vi "Get Data Name from TD__ogtk.vi"(8 "error in (no error)":errorcluster, 10 "Type Descriptor":T1) -> (0 "error":errorcluster, 2 "name":string)   [LabVIEW 2020, in "openg_variant.lvlib"]
doc: "Returns the name of the data described by the type string input."
uses:
  openg_variant.lvlib
  Type Descriptor__ogtk.ctl
  openg_error.lvlib
panel:
  # "[OpenG VI Tags] ***Do Not Remove***"
  # "Get Data Name from TD.vi\n\nReturns the name of the data described by the type string input.\n\nPlease visit http://www.OpenG.org to learn about the\nOpen Source LabVIEW software movement.\n\nNOTICE -- YOU MUST LEAVE THIS NOTICE IN PLACE.  PER THE TERMS OF THE LICENSE BELOW, YOU MAY SUBLICENSE THIS SOFTWARE \nIN ANY WAY THAT DOES NOT CONFLICT WITH THIS LICENSE.\n\n### BSD License (http://www.opensource.org/licenses/bsd-license.php) Begin ###\n \nCopyright (c) 2002, Jean-Pierre Drolet <drolet_jp@hotmail.com>\nCopyright (c) 2002-2006, Jim Kring <jim@jimkring.com>\n\nAll rights reserved.\n\nRedistribution and use in source and binary forms, with or without modification, are permitted provided that the following conditions are met:\n\n    * Redistributions of source code must retain the above copyright notice, this list of conditions and the following disclaimer.\n    * Redistributions in binary form must reproduce the above copyright notice, this list of conditions and the following disclaimer in the \n       documentation and/or other materials provided with the distribution.\n    * Neither the name of SciWare, James Kring, Inc., nor the names of its contributors may be used to endorse or promote products derived \n       from this software without specific prior written permission.\n\nTHIS SOFTWARE IS PROVIDED BY THE COPYRIGHT HOLDERS AND CONTRIBUTORS \"AS IS\" AND ANY EXPRESS OR IMPLIED WARRANTIES, \nINCLUDING, BUT NOT LIMITED TO, THE IMPLIED WARRANTIES OF MERCHANTABILITY AND FITNESS FOR A PARTICULAR PURPOSE ARE \nDISCLAIMED. IN NO EVENT SHALL THE COPYRIGHT OWNER OR CONTRIBUTORS BE LIABLE FOR ANY DIRECT, INDIRECT, INCIDENTAL,\n SPECIAL, EXEMPLARY, OR CONSEQUENTIAL DAMAGES (INCLUDING, BUT NOT LIMITED TO, PROCUREMENT OF SUBSTITUTE GOODS OR \nSERVICES; LOSS OF USE, DATA, OR PROFITS; OR BUSINESS INTERRUPTION) HOWEVER CAUSED AND ON ANY THEORY OF LIABILITY, \nWHETHER IN CONTRACT, STRICT LIABILITY, OR TORT (INCLUDING NEGLIGENCE OR OTHERWISE) ARISING IN ANY WAY OUT OF THE USE \nOF THIS SOFTWARE, EVEN IF ADVISED OF THE POSSIBILITY OF SUCH DAMAGE.\n\n### BSD License End ###"
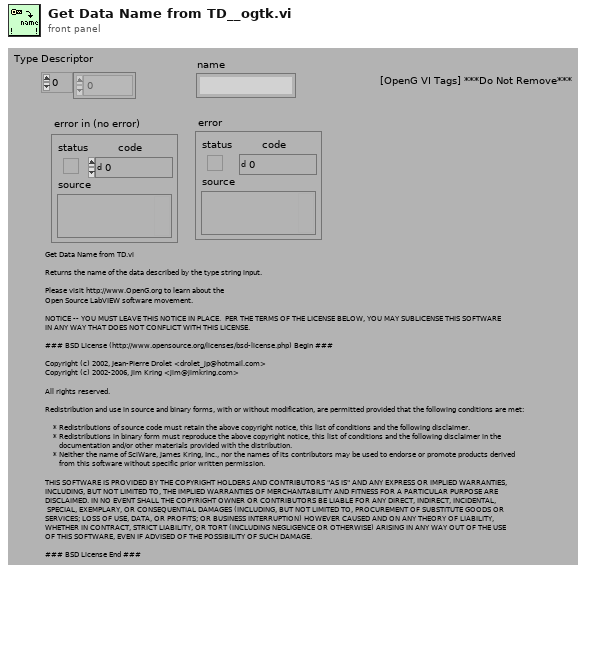
[diagram p1: front panel]
types:
  T1 = typedef "openg_variant.lvlib/Type Descriptor__ogtk.ctl" = i16[]
  T2 = typedef "openg_variant.lvlib/Type Descriptor Header__ogtk.ctl" = cluster{"length":u16, "private":u8, "type":T3, "# elements":u16}
  T3 = typedef "openg_variant.lvlib/Type Descriptor Enumeration__ogtk.ctl" = enum8{"<Null>", "I8", "I16", "I32", "I64", "U8", "U16", "U32", "U64", "SGL", "DBL", "EXT", "CSG", "CDB", "CXT", "0x0F", "0x10", "0x11", "0x12", "0x13", "0x14", "Enum U8", "Enum U16", "Enum U32", "Enum U64", "SGL PQ", "DBL PQ", "EXT PQ", "CSG PQ", "CDB PQ", "CXT PQ", "0x1F", "0x20", "Boolean", "0x22", "0x23", "0x24", "0x25", "0x26", "0x27", "0x28", "0x29", "0x2A", "0x2B", "0x2C", "0x2D", "0x2E", "0x2F", "String", "0x31", "Path", "Pict", "0x34", "0x35", "0x36", "DAQ", "0x38", "0x39", "0x3A", "0x3B", "0x3C", "0x3D", "0x3E", "0x3F", "Array", "0x41", "0x42", "0x43", "0x44", "0x45", "0x46", "0x47", "0x48", "0x49", "0x4A", "0x4B", "0x4C", "0x4D", "0x4E", "0x4F", "Cluster", "0x51", "0x52", "Variant", "Waveform", "0x55", "0x56", "0x57", "0x58", "0x59", "0x5A", "0x5B", "0x5C", "0x5D", "0x5E", "Fixed Point", "0x60", "0x61", "0x62", "0x63", "0x64", "0x65", "0x66", "0x67", "0x68", "0x69", "0x6A", "0x6B", "0x6C", "0x6D", "0x6E", "0x6F", "Refnum", "0x71", "0x72", "Set Collection", "Map Collection"}
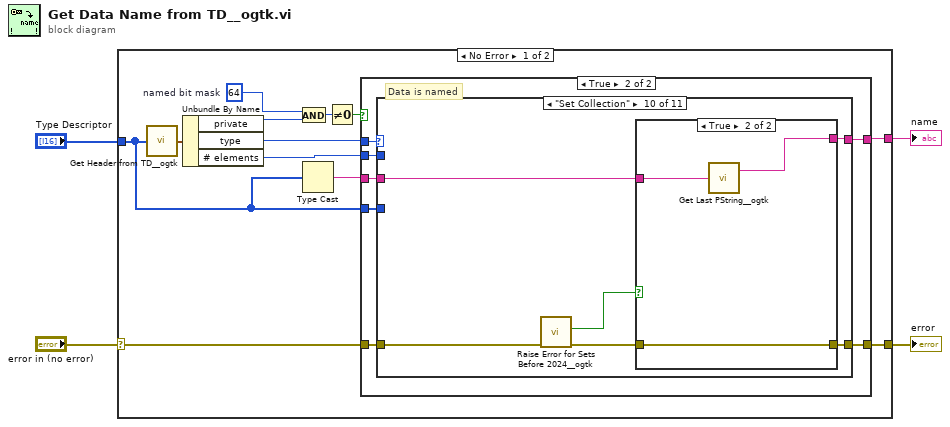
[diagram p0: block diagram]
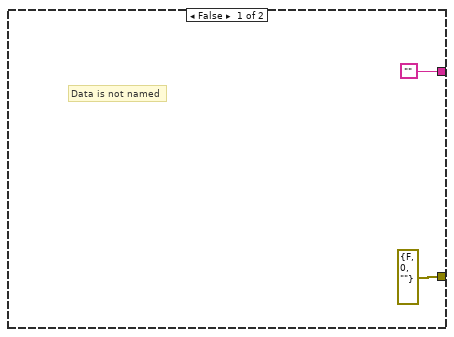
[diagram p2: hidden frame]
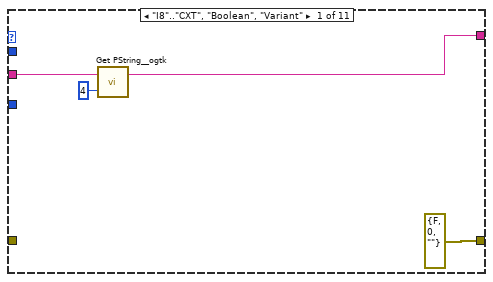
[diagram p3: hidden frame]
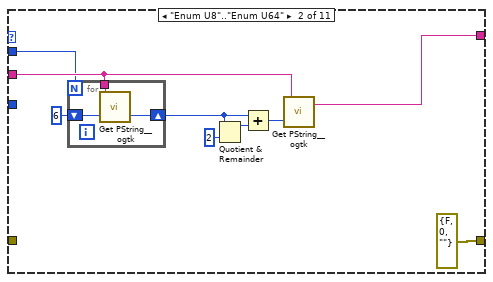
[diagram p4: hidden frame]
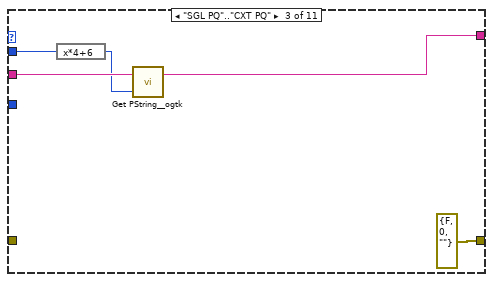
[diagram p5: hidden frame]
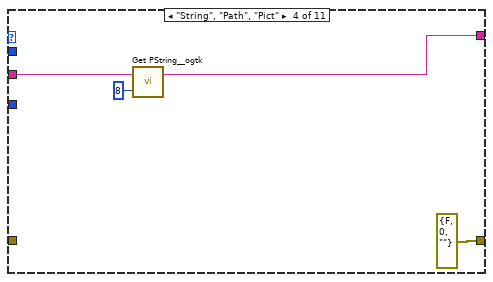
[diagram p6: hidden frame]
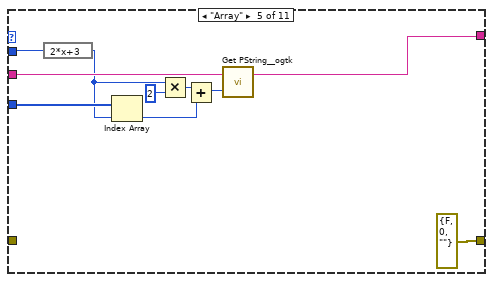
[diagram p7: hidden frame]
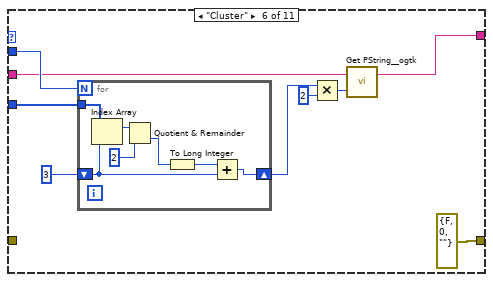
[diagram p8: hidden frame]
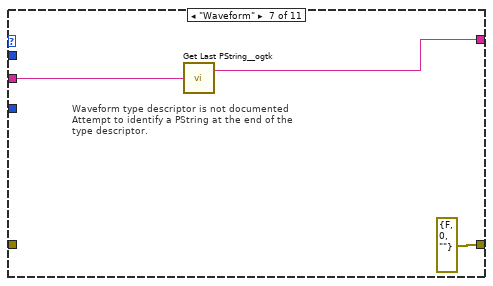
[diagram p9: hidden frame]
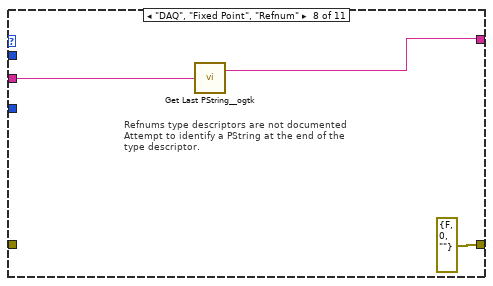
[diagram p10: hidden frame]
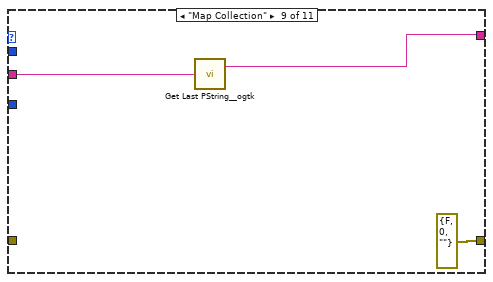
[diagram p11: hidden frame]
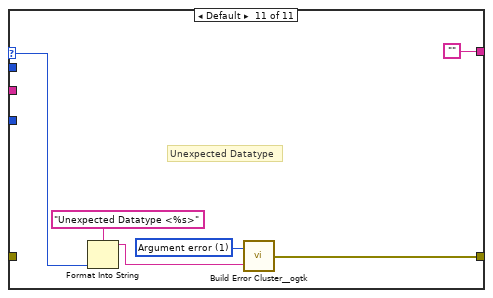
[diagram p13: hidden frame]
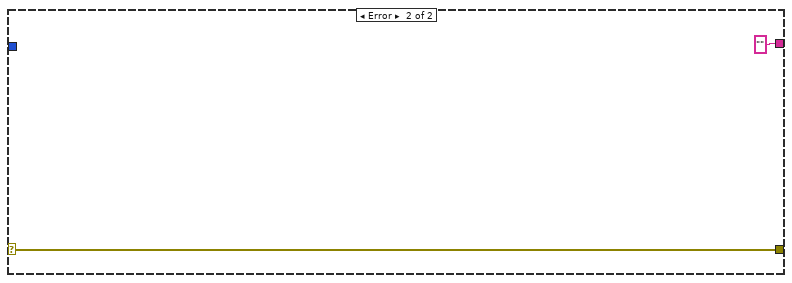
[diagram p14: hidden frame]
diagram:
  n1 = case shown="No Error" "error in (no error)" {
    selector: "error in (no error)" -> [w5 w103]
    tunnel: "Type Descriptor" -> [w15 _]
    tunnel: [w12 "" ("Last PString")] -> w3
    tunnel: [w6 w103] -> w2
    frame No Error {
      w9 = u8 64  # named bit mask
      n2 = call "Get Header from TD__ogtk.vi"("Type Descriptor"=w15) -> ("Type Descriptor Header"=w16:T2)
      n3 = Unbundle By Name(w16) -> ("private"=w8:u8, "type"=w7:T3, "# elements"=w14:u16)
      n4 = And(x=w9, y=w8) -> (x .and. y?=w11:u8)
      n5 = Type Cast(x=w15) -> (*(type *) &x=w13:string)  [unwired: 1 in]
      n6 = Not Equal To 0?(x=w11) -> (x != 0?=w10:bool)
      n7 = case shown="True" w10 {
        tunnel: [errorcluster {"status"=FALSE, "code"=0, "source"=""} ("error out") w25] -> w6
        tunnel: w7 -> [_ w24]
        tunnel: w13 -> [_ w23]
        tunnel: ["" w22] -> w12
        tunnel: w14 -> [_ w21]
        tunnel: w15 -> [_ w20]
        tunnel: w5 -> [_ w19]
        frame False {
          # "Data is not named"
        }
        frame True {
          # "Data is named"
          n8 = case shown="\"Set Collection\"" w24 {
            selector: w24 -> [_ _ _ _ _ _ _ _ _ _ w96]
            tunnel: [errorcluster {"status"=FALSE, "code"=0, "source"=""} ("error out") errorcluster {"status"=FALSE, "code"=0, "source"=""} ("error out") errorcluster {"status"=FALSE, "code"=0, "source"=""} ("error out") errorcluster {"status"=FALSE, "code"=0, "source"=""} ("error out") errorcluster {"status"=FALSE, "code"=0, "source"=""} ("error out") errorcluster {"status"=FALSE, "code"=0, "source"=""} ("error out") errorcluster {"status"=FALSE, "code"=0, "source"=""} ("error out") errorcluster {"status"=FALSE, "code"=0, "source"=""} ("error out") errorcluster {"status"=FALSE, "code"=0, "source"=""} ("error out") w89 w101] -> w25
            tunnel: w23 -> [w28 w35 w45 w50 w57 w66 w78 w82 w85 w91 _]
            tunnel: [w26 w34 w43 w49 w56 w65 w77 w81 w84 w90 ""] -> w22
            tunnel: w21 -> [_ w32 w46 _ w59 w68 _ _ _ _ _]
            tunnel: w20 -> [_ _ _ _ w58 w67 _ _ _ _ _]
            tunnel: w19 -> [_ _ _ _ _ _ _ _ _ w87 _]
            frame "I8".."CXT", "Boolean", "Variant" {
              n9 = call "Get PString__ogtk.vi"("offset (0)"=4, "String"=w28) -> ("PString"=w26:string)  [unwired: 1 out]
            }
            frame "Enum U8".."Enum U64" {
              n10 = for {
                N: w32 -> [_]
                tunnel: w35 -> [w39]
                shift-right: [w40] -> w37
                shift-left: 6 -> [w41]
                n11 = call "Get PString__ogtk.vi"("offset (0)"=w41, "String"=w39) -> ("offset past PString"=w40:i32)  [unwired: 1 out]
              }
              n12 = Quotient & Remainder(x=w37, y=2) -> (x-y*floor(x/y)=w30:i32)  [unwired: 1 out]
              n13 = Add(x=w37, y=w30) -> (x+y=w36:i32)
              n14 = call "Get PString__ogtk.vi"("offset (0)"=w36, "String"=w35) -> ("PString"=w34:string)  [unwired: 1 out]
            }
            frame "SGL PQ".."CXT PQ" {
              n15 = expression code="x*4+6"(w46) -> (w44:u16)
              n16 = call "Get PString__ogtk.vi"("offset (0)"=w44, "String"=w45) -> ("PString"=w43:string)  [unwired: 1 out]
            }
            frame "String", "Path", "Pict" {
              n17 = call "Get PString__ogtk.vi"("offset (0)"=8, "String"=w50) -> ("PString"=w49:string)  [unwired: 1 out]
            }
            frame "Array" {
              n18 = expression code="2*x+3"(w59) -> (w55:u16)
              n19 = Index Array(array=w58, index=w55) -> (element=w52:i16)
              n20 = Multiply(x=w55, y=u16 2) -> (x*y=w53:u16)
              n21 = Add(x=w53, y=w52) -> (x+y=w51:u16)
              n22 = call "Get PString__ogtk.vi"("offset (0)"=w51, "String"=w57) -> ("PString"=w56:string)  [unwired: 1 out]
            }
            frame "Cluster" {
              n23 = for {
                N: w68 -> [_]
                shift-right: [w75] -> w63
                shift-left: 3 -> [w74]
                tunnel: w67 -> [w76]
                n24 = Index Array(array=w76, index=w74) -> (element=w72:i16)
                n25 = Quotient & Remainder(x=w72, y=i16 2) -> (floor(x/y)=w73:i16)  [unwired: 1 out]
                n26 = To Long Integer(number=w73) -> (32bit integer=w70:i32)
                n27 = Add(x=w70, y=w74) -> (x+y=w75:i32)
              }
              n28 = Multiply(x=w63, y=2) -> (x*y=w62:i32)
              n29 = call "Get PString__ogtk.vi"("offset (0)"=w62, "String"=w66) -> ("PString"=w65:string)  [unwired: 1 out]
            }
            frame "Waveform" {
              # "Waveform type descriptor is not documented\nAttempt to identify a PString at the end of the\ntype descriptor."
              n30 = call "Get Last PString__ogtk.vi"("String"=w78) -> ("Last PString"=w77:string)  [unwired: 1 out]
            }
            frame "DAQ", "Fixed Point", "Refnum" {
              # "Refnums type descriptors are not documented\nAttempt to identify a PString at the end of the\ntype descriptor."
              n31 = call "Get Last PString__ogtk.vi"("String"=w82) -> ("Last PString"=w81:string)  [unwired: 1 out]
            }
            frame "Map Collection" {
              n32 = call "Get Last PString__ogtk.vi"("String"=w85) -> ("Last PString"=w84:string)  [unwired: 1 out]
            }
            frame "Set Collection" {
              n33 = call "Raise Error for Sets Before 2024__ogtk.vi"("error in (no error)"=w87) -> ("error out"=w86:errorcluster, "supported?"=w88:bool)  [unwired: 9 in]
              n34 = case shown="True" w88 {
                tunnel: w91 -> [_ w95]
                tunnel: [_ w94] -> w90
                tunnel: [w92 w93] -> w89
                tunnel: w86 -> [w92 w93]
                frame False {
                }
                frame True {
                  n35 = call "Get Last PString__ogtk.vi"("String"=w95) -> ("Last PString"=w94:string)  [unwired: 1 out]
                }
              }
            }
            frame Default {
              w100 = 1 items=["No error", "Argument error", "Memory is full", "Out of zone", "End of file", "File already open", "Generic file I/O error", "File not found", "File permission error", "Disk is full", "Duplicate path", "Too many files open", "System feature not enabled", "Resource file not found", "Cannot add resource", "Resource not found", "Image not found", "Image memory error", "Pen does not exist", "Config type invalid", "Config token not found", "Config parse error", "Config memory error", "Bad external code format", "Bad external code offset", "External code not present", "Null window", "Destroy window error", "Null menu", "Print aborted", "Bad print record", "Print driver error", "Windows error during printing", "Memory error during printing", "Print dialog error", "Generic print error", "Invalid device refnum", "Device not found", "Device parameter error", "Device unit error", "Cannot open device", "Device call aborted", "Generic error", "Cancelled by user", "Object ID too low", "Object ID too high", "Object not in heap", "Unknown heap", "Unknown object (invalid DefProc)", "Unknown object (DefProc not in table)", "Message out of range", "Invalid (null) method", "Unknown message", "Manager call not supported", "Bad address", "Network operation in progress", "Network operation timed out", "Connection is busy", "Network attribute not supported", "Network error", "Address in use", "System out of memory", "Connection aborted", "Connection refused", "Not connected", "Already connected", "Connection closed", "Initialization error (interapplication manager)", "Bad occurrence", "Wait on unbound occurrence handler", "Occurrence queue overflow", "Datalog type conflict", "Unused", "Unrecognized type (interapplication manager)", "Memory corrupt", "Failed to make temporary DLL", "Old CIN version", "Drag socket not found", "Failed to load drop-object", "Failed to register OLE object", "Failed to release OLE object", "Format specifier type mismatch", "Unknown format specifier", "Too few format specifiers", "Too many format specifiers", "Scan failed", "Newer CIN version", "Error converting to variant", "Runtime menu error", "Password tampered", "Variant attribute not found", "Incompatible variant data type", "Event data is not available", "Event Store is not present", "Occurrence is not found", "Event Queue is not created", "Event info is not available", "Refnum passed is NULL", "Error retrieving Class GUID", "Error retrieving CoClass GUID", "Error retrieving TypeLib GUID.", "Bad built application magic bytes.", "Specific driver is different from the specific driver associated with the Logical Name.", "There is no session opened to the class driver.", "Max Error", "MAX - Error with config objects", "MAX - Error loading configuration", "MAX - Group not supported"]
              # "Unexpected Datatype"
              n36 = Format Into String(format string="Unexpected Datatype <%s>" ("Format String"), w96) -> (resulting string=w97:string)  [unwired: 2 in, 1 out]
              n37 = call "Build Error Cluster__ogtk.vi"("String to Prepend to source (\"\")"=w97, "code"=w100) -> ("error out"=w101:errorcluster)
            }
          }
        }
      }
    }
    frame Error {
    }
  }
  "name" <- w3
  "error" <- w2
